vi "Decode Parameter (DBL) from Word.vi"(8 "error in":errorcluster, 9 "parameter definition":T1, 11 "32-bit word in":u32 format="%032b") -> (0 "error out":errorcluster, 2 "parameter value":dbl, 3 "32-bit word out":u32 format="%032b")   [LabVIEW 2020]
uses:
  Parameter Definition.ctl
  <vilib>/NI/NI VeriStand Encoding and Decoding/Encoding.ctl
  1980749b-e417-4a21-943a-7c30016504b0.vi
  1f3c3557-5c17-491c-9e18-ef0b55369bc3.vi
  1980749b-e417-4a21-943a-7c30016504b0.vi/16a2565b-3c16-407b-a626-9da2a3da432e.vi
  1f3c3557-5c17-491c-9e18-ef0b55369bc3.vi/0a001d06-2809-4638-8d0b-e017d2157007.vi
  1f3c3557-5c17-491c-9e18-ef0b55369bc3.vi/e08d08e5-79bf-42ec-a5e5-c4db927cd1a5.vi
  1f3c3557-5c17-491c-9e18-ef0b55369bc3.vi/e1d6a9f9-c3bf-4c4f-a94d-c7d44a3a2cb5.vi
  <vilib>/NI/NI VeriStand Encoding and Decoding/Get Bits Per Digit from Base.vi
  <vilib>/NI/NI VeriStand Encoding and Decoding/Encoding and Decoding.lvlib
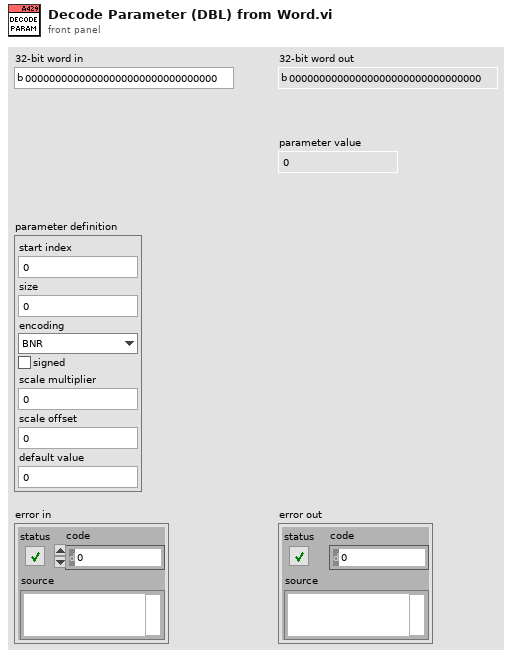
[diagram p1: front panel]
types:
  T1 = typedef "Parameter Definition.ctl" = cluster{"start index":i32, "size":i32, "encoding":T2, "signed":bool, "scale multiplier":dbl, "scale offset":dbl, "default value":dbl}
  T2 = typedef "Encoding and Decoding.lvlib/Encoding.ctl" = enum16{"BNR", "BCD", "Discrete"}
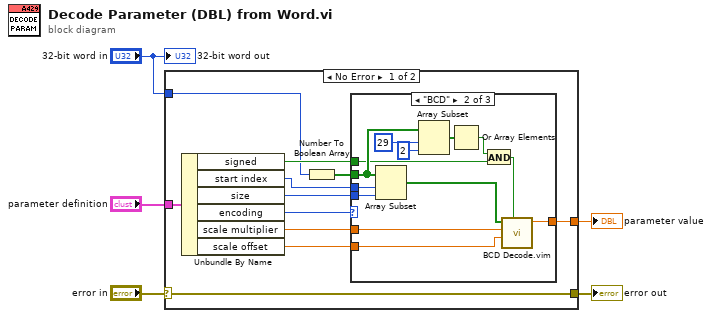
[diagram p0: block diagram]
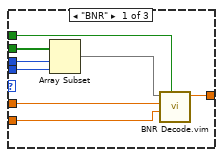
[diagram p2: hidden frame]
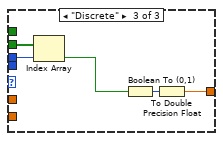
[diagram p3: hidden frame]
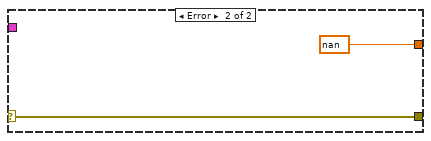
[diagram p4: hidden frame]
diagram:
  n1 = case shown="No Error" "error in" {
    selector: "error in" -> [w6 w44]
    tunnel: [w12 nan ("value")] -> w3
    tunnel: "32-bit word in" -> [w11 _]
    tunnel: "parameter definition" -> [w10 _]
    tunnel: [w6 w44] -> w2
    frame No Error {
      n2 = Unbundle By Name(w10) -> ("signed"=w13:bool, "start index"=w15:i32, "size"=w16:i32, "encoding"=w7:T2, "scale multiplier"=w8:dbl, "scale offset"=w9:dbl)
      n3 = Number To Boolean Array(number=w11) -> (Boolean array=w14:bool[])
      n4 = case shown="\"BCD\"" w7 {
        tunnel: w8 -> [w24 w36 _]
        tunnel: w9 -> [w23 w35 _]
        tunnel: w13 -> [w22 w25 _]
        tunnel: [w21 w37 w38] -> w12
        tunnel: w14 -> [w20 w31 w42]
        tunnel: w15 -> [w19 w34 w41]
        tunnel: w16 -> [w18 w33 _]
        frame "BNR" {
          n5 = Array Subset(array=w20, index=w19, length=w18) -> (w17:bool[])
          n6 = call "BNR Decode.vim"("signed"=w22, "scale offset"=w23, "scale multiplier"=w24, "BNR encoded value"=w17) -> ("value"=w21:dbl)  [unwired: 7 in]
        }
        frame "BCD" {
          n7 = Array Subset(array=w31, index=w34, length=w33) -> (w32:bool[])
          n8 = Array Subset(array=w31, index=29, length=2) -> (w28:bool[])
          n9 = Or Array Elements(Boolean array=w28) -> (logical OR=w27:bool)
          n10 = And(x=w27, y=w25) -> (x .and. y?=w26:bool)
          n11 = call "BCD Decode.vim"("signed"=w26, "scale offset"=w35, "scale multiplier"=w36, "BCD encoded value"=w32) -> ("value"=w37:dbl)  [unwired: 7 in]
        }
        frame "Discrete" {
          n12 = Index Array(array=w42, index=w41) -> (element=w40:bool)
          n13 = Boolean To (0,1)(Boolean=w40) -> (0, 1=w39:i16)
          n14 = To Double Precision Float(number=w39) -> (double precision float=w38:dbl)
        }
      }
    }
    frame Error {
    }
  }
  "error out" <- w2
  "parameter value" <- w3
  "32-bit word out" <- "32-bit word in"
